vi "Get Filter Name Array.vi"(11 "Main Display in":refnum<class "Main Display.lvclass">) -> (2 "Filter Name Array":string[](array[string]))   [LabVIEW 2016, in "Assert API Components.lvlib" / "Assert Display.lvlib" / "Main Display.lvlib" / "Main Display.lvclass"]
uses:
  Core/Main Display/Main Display/Main Display.lvclass
  Core/Main Display/Main Display/Main Display.lvclass/Main Display.ctl
  Core/Assert API Components/Filter Configurations/Base Filter.lvclass/Base Filter.ctl
  Core/Assert API Components/Filter Configurations/Base Filter.lvclass
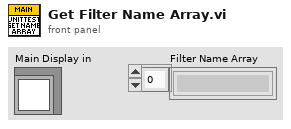
[diagram p1: front panel]
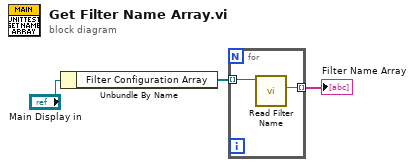
[diagram p0: block diagram]
diagram:
  n1 = Unbundle By Name("Main Display in") -> ("Filter Configuration Array"=w2:refnum<class "Base Filter.lvclass">[])
  n2 = for {
    tunnel: w2 -> [w5] mode=indexing
    tunnel: [w4] -> w3 mode=indexing
    n3 = call "Read Filter Name.vi"("Base Filter in"=w5) -> ("Filter Name"=w4:string)  [unwired: 10 in]
  }
  "Filter Name Array" <- w3
